vi "push_model.vi"() -> ()   [LabVIEW 2013]
uses:
  GlobleVar/segment_size.vi
  GlobleVar/Data.vi
panel:
  out "size(s)":i32[](array[numeric])
  in  "stop":bool
  out "Array":dbl[][](array[numeric])
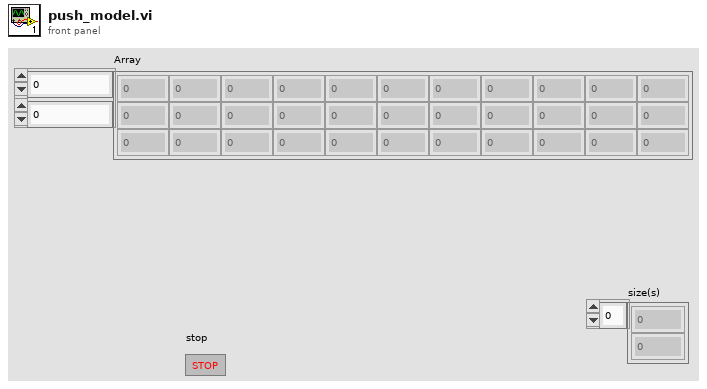
[diagram p1: front panel]
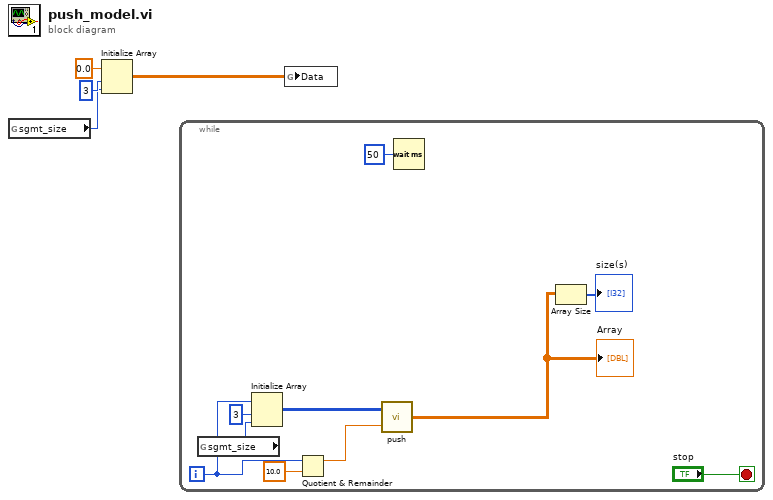
[diagram p0: block diagram]
diagram:
  n1 = global read "segment_size.vi" "sgmt_size"() -> (w1:i32)
  n2 = Initialize Array(0.0 ("element"), 3 ("dimension size"), w1) -> (w2:dbl[][])
  n3 = while {
    i -> [w10]
    stop <- "stop" stop-if-true
    n4 = global read "segment_size.vi" "sgmt_size"() -> (w7:i32)
    n5 = Initialize Array(w10, 3 ("dimension size"), w7) -> (w9:i32[][])
    n6 = Quotient & Remainder(x=w10, y=10.0) -> (x-y*floor(x/y)=w8:dbl)  [unwired: 1 out]
    n7 = call "push.vi"("ptr_write"=w8, "Data in"=w9) -> ("Data"=w6:dbl[][])
    "Array" <- w6
    n8 = Wait (ms)(milliseconds to wait=u32 50) -> ()  [unwired: 1 out]
    n9 = Array Size(array=w6) -> (size(s)=→"size(s)":i32[])
  }
  n10 = global write "Data.vi" "Data"(w2) -> ()
